vi "Update Bounds.vi"(8 "error in (no error)":errorcluster, 10 "Bounds":T1, 11 "GUI Helper in":refnum<class "GUI Helper.lvclass">) -> (0 "error out":errorcluster, 3 "GUI Helper out":refnum<class "GUI Helper.lvclass">)   [LabVIEW 2020, in "VolatusGUI.lvlib" / "GUI Helper.lvclass"]
uses:
  GUI Helper.lvclass
  <vilib>/Utility/miscctls.llb/LVRectTypeDef.ctl
  Position Data.ctl
  GUI Helper.lvclass/GUI Helper.ctl
  Volatus/MessageQ/MessageQ.lvclass/MessageQ.ctl
  Volatus/MessageQ/MessageQ.lvclass
  VolatusGUI.lvlib
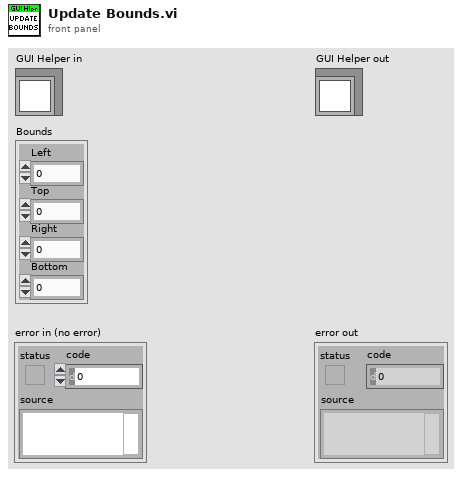
[diagram p1: front panel]
types:
  T1 = typedef "LVRectTypeDef.ctl" = cluster{"Left":i16, "Top":i16, "Right":i16, "Bottom":i16}
  T2 = typedef "VolatusGUI.lvlib/Position Data.ctl" = cluster{"GUI ID":string, "Bounds":T1}
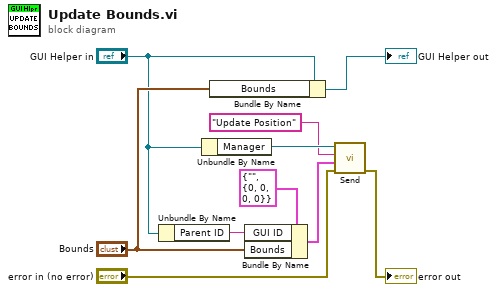
[diagram p0: block diagram]
diagram:
  n1 = Unbundle By Name("GUI Helper in") -> ("Parent ID"=w1:string)
  n2 = Unbundle By Name("GUI Helper in") -> ("Manager"=w10:refnum<class "MessageQ.lvclass">)
  n3 = Bundle By Name(cluster="GUI Helper in", "Bounds"="Bounds") -> (→"GUI Helper out":refnum<class "GUI Helper.lvclass">)
  n4 = Bundle By Name(cluster=T2 {"GUI ID"="", "Bounds"={"Left"=0, "Top"=0, "Right"=0, "Bottom"=0}} ("Position Message"), "GUI ID"=w1, "Bounds"="Bounds") -> (w7:T2)
  n5 = call "Send.vi"("error in (no error)"="error in (no error)", "Data"=w7, "ID"="Update Position", "MessageQ in"=w10) -> ("error out"=→"error out":errorcluster)  [unwired: 6 in, 1 out]
